vi "write_corr_coeff.vi"(0 "C\n(Ax^2+Bx+C)":dbl=360.60296, 1 "B\n(Ax^2+Bx+C)":dbl=0.13277, 2 "A\n(Ax^2+Bx+C)":dbl=5.88212e-06, 3 "bck: b\n(ax+b)":dbl, 4 "bck: a\n(ax+b)":dbl) -> (5 "Write array":u8[](array[numeric]))   [LabVIEW 2022 SP3]
panel:
  out "size(s)":i32
  in  "additional info 16":string="LR2 4.0 c.N 0604"
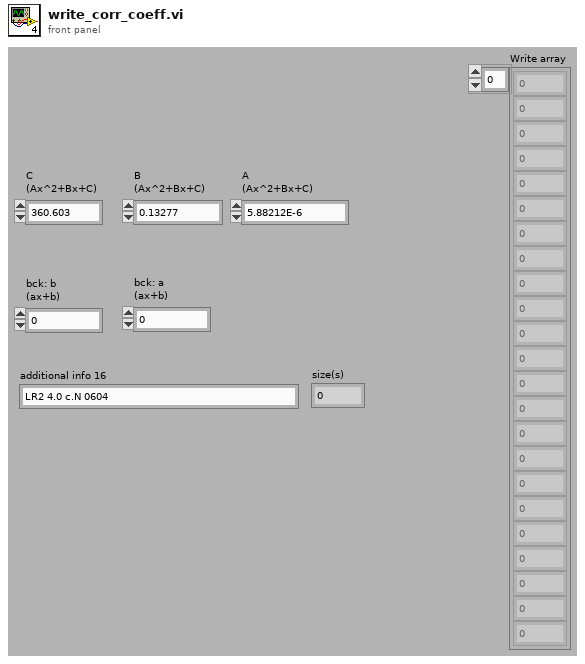
[diagram p1: front panel]
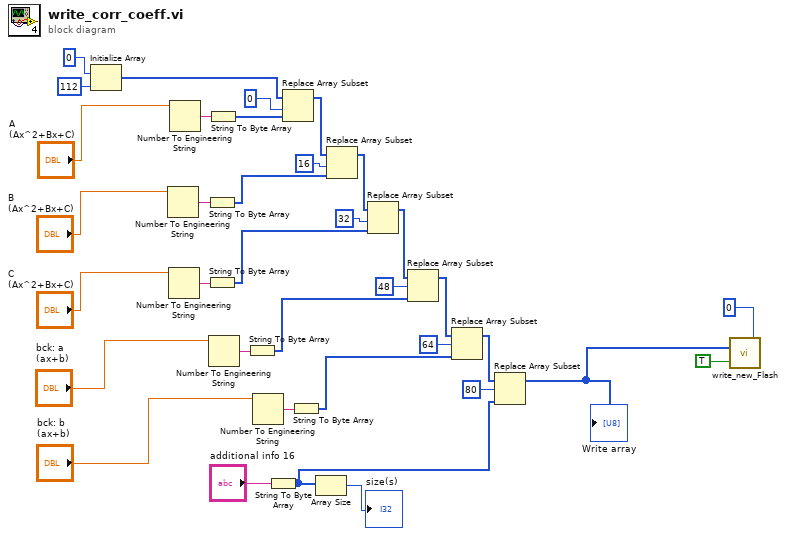
[diagram p0: block diagram]
diagram:
  n1 = Initialize Array(u8 0, 112 ("dimension size")) -> (w27:u8[])
  n2 = Number To Engineering String(4:"B\n(Ax^2+Bx+C)") -> (0:w29:string)  [unwired: 3 in]
  n3 = Number To Engineering String(4:"C\n(Ax^2+Bx+C)") -> (0:w28:string)  [unwired: 3 in]
  n4 = Number To Engineering String(4:"A\n(Ax^2+Bx+C)") -> (0:w30:string)  [unwired: 3 in]
  n5 = String To Byte Array(string=w29) -> (unsigned byte array=w23:u8[])
  n6 = String To Byte Array(string=w28) -> (unsigned byte array=w20:u8[])
  n7 = String To Byte Array(string=w30) -> (unsigned byte array=w26:u8[])
  n8 = Number To Engineering String(4:"bck: a\n(ax+b)") -> (0:w18:string)  [unwired: 3 in]
  n9 = String To Byte Array(string=w18) -> (unsigned byte array=w17:u8[])
  n10 = Number To Engineering String(4:"bck: b\n(ax+b)") -> (0:w14:string)  [unwired: 3 in]
  n11 = String To Byte Array(string="additional info 16") -> (unsigned byte array=w2:u8[])
  n12 = Replace Array Subset(array=w27, new element=w26, index=0) -> (w24:u8[])
  n13 = String To Byte Array(string=w14) -> (unsigned byte array=w13:u8[])
  n14 = Array Size(array=w2) -> (size(s)=→"size(s)":i32)
  n15 = Replace Array Subset(array=w24, new element=w23, index=16) -> (w21:u8[])
  n16 = Replace Array Subset(array=w21, new element=w20, index=32) -> (w15:u8[])
  n17 = Replace Array Subset(array=w15, new element=w17, index=48) -> (w11:u8[])
  n18 = Replace Array Subset(array=w11, new element=w13, index=64) -> (w5:u8[])
  n19 = Replace Array Subset(array=w5, new element=w2, index=80) -> (w4:u8[])
  "Write array" <- w4
  n20 = call "write_new_Flash.vi"("address (3 bytes)"=u32 0, "sector erase"=TRUE, "write array"=w4) -> ()
